vi "차선인식2subVI.vi"(0 "Image In":T9, 1 "Color Mode (Color Threshold 1)":u16(ring) items=["RGB", "HSL", "HSV", "HSI"], 2 "Red or Hue Range (Color Threshold 1)":cluster{"Lower value":i32, "Upper value":i32}={"Lower value"=17, "Upper value"=214}, 3 "Green or Sat Range (Color Threshold 1)":cluster{"Lower value":i32, "Upper value":i32}={"Lower value"=35, "Upper value"=255}, 4 "Blue or Luma or Val or Inten Range (Color Threshold 1)":cluster{"Lower value":i32, "Upper value":i32}={"Lower value"=38, "Upper value"=178}, 5 "Filter Parameters (Filters 1)":T5={"Sigma"=2.0, "HThresh"=0.95, "LThres"=0.8, "WindowSize"=7}, 6 "Operation (Gray Morphology 1)":T4(ring)=enum."Dilate", 7 "error in":errorcluster, 8 "Structuring Element (Gray Morphology 1)":i32[][](array[numeric])=[[1, 1, 1], [1, 1, 1], [1, 1, 1]], 9 "ROI Descriptor (Adv. Straight Edge 1)":T3={"Global Rectangle"=[36, 66, 280, 304], "Contours"=[{"ID"=enum."External", "Type"=12, "Coordinates"=[117, 56, 199, 314, 313366]}]} {"Contours"."Type" items=["No Selection", "Point", "Line", "Rectangle", "Oval", "Polygon", "Freehand Region", "Annulus", "Unused2", "Unused3", "Broken Line", "Freehand Line", "Rotated Rectangle"]}, 10 "Edge Options (Adv. Straight Edge 1)":T2={"Edge Polarity"=1, "Kernel Size"=13, "Width"=3, "Minimum Edge Strength"=26.34, "Interpolation Type"=enum."Zero Order", "Data Processing Method"=enum."Average"} {"Edge Polarity" items=["All Edges", "Rising Edges", "Falling Edges"]}, 11 "Search Direction (Adv. Straight Edge 1)":u32(ring)=1 items=["Left to Right", "Right to Left", "Top to Bottom", "Bottom to Top"], 12 "Line Options (Adv. Straight Edge 1)":T1={"Number of Lines"=1, "Type"=enum."Best Edge Projection", "Min. Score"=0.0, "Max. Score"=1024.0, "Orientation"=0.0, "Angle Range"=20.0, "Angle Tolerance"=1.0, "Step Size"=12, "Min. SNR (db)"=0.0, "Min. Points (%)"=25.0, "Hough Iterations"=5}, 13 "ROI Descriptor (Adv. Straight Edge 2)":T3={"Global Rectangle"=[252, 97, 418, 305], "Contours"=[{"ID"=enum."External", "Type"=12, "Coordinates"=[296, 104, 374, 298, 30219]}]} {"Contours"."Type" items=["No Selection", "Point", "Line", "Rectangle", "Oval", "Polygon", "Freehand Region", "Annulus", "Unused2", "Unused3", "Broken Line", "Freehand Line", "Rotated Rectangle"]}, 14 "Edge Options (Adv. Straight Edge 2)":T2={"Edge Polarity"=1, "Kernel Size"=7, "Width"=3, "Minimum Edge Strength"=122.7, "Interpolation Type"=enum."Zero Order", "Data Processing Method"=enum."Average"} {"Edge Polarity" items=["All Edges", "Rising Edges", "Falling Edges"]}, 15 "Search Direction (Adv. Straight Edge 2)":u32(ring) items=["Left to Right", "Right to Left", "Top to Bottom", "Bottom to Top"], 16 "Line Options (Adv. Straight Edge 2)":T1={"Number of Lines"=1, "Type"=enum."Best Edge Projection", "Min. Score"=0.0, "Max. Score"=1024.0, "Orientation"=0.0, "Angle Range"=20.0, "Angle Tolerance"=1.0, "Step Size"=31, "Min. SNR (db)"=0.0, "Min. Points (%)"=25.0, "Hough Iterations"=5}) -> (20 "Image Out":T9, 21 "Straight Edges (Adv. Straight Edge 1)":T7(array[cluster]) {"Point2 (Real-World)"."Y" format="%.2f"; "Point2 (Real-World)"."X" format="%.2f"; "Point1 (Real-World)"."Y" format="%.2f"; "Point1 (Real-World)"."X" format="%.2f"; "Point2 (Pixels)"."Y" format="%.2f"; "Point2 (Pixels)"."X" format="%.2f"; "Point1 (Pixels)"."Y" format="%.2f"; "Point1 (Pixels)"."X" format="%.2f"}, 22 "Search Lines Information (Adv. Straight Edge 1)":T8(array[cluster]) {"Edges"."Distance (Real-World)" format="%.2f"; "Edges"."Location (Real-World)"."Y" format="%.2g"; "Edges"."Location (Real-World)"."X" format="%.2f"; "Edges"."Noise" format="%.2f"; "Edges"."Location (Pixel)"."Y" format="%.2g"; "Edges"."Location (Pixel)"."X" format="%.2f"; "Edges"."Strength" format="%.2f"; "Edges"."Distance (Pixel)" format="%.2f"; "End Point"."Y" format="%.2f"; "End Point"."X" format="%.2f"; "Start Point"."Y" format="%.2f"; "Start Point"."X" format="%.2f"}, 23 "Used Edges (Adv. Straight Edge 1)":cluster{"Edge Information":T6[]}[](array[cluster]) {"Edge Information"."Distance (Real-World)" format="%.2f"; "Edge Information"."Location (Real-World)"."Y" format="%.2g"; "Edge Information"."Location (Real-World)"."X" format="%.2f"; "Edge Information"."Noise" format="%.2f"; "Edge Information"."Location (Pixel)"."Y" format="%.2g"; "Edge Information"."Location (Pixel)"."X" format="%.2f"; "Edge Information"."Strength" format="%.2f"; "Edge Information"."Distance (Pixel)" format="%.2f"}, 24 "Straight Edges (Adv. Straight Edge 2)":T7(array[cluster]) {"Point2 (Real-World)"."Y" format="%.2f"; "Point2 (Real-World)"."X" format="%.2f"; "Point1 (Real-World)"."Y" format="%.2f"; "Point1 (Real-World)"."X" format="%.2f"; "Point2 (Pixels)"."Y" format="%.2f"; "Point2 (Pixels)"."X" format="%.2f"; "Point1 (Pixels)"."Y" format="%.2f"; "Point1 (Pixels)"."X" format="%.2f"}, 25 "Search Lines Information (Adv. Straight Edge 2)":T8(array[cluster]) {"Edges"."Distance (Real-World)" format="%.2f"; "Edges"."Location (Real-World)"."Y" format="%.2g"; "Edges"."Location (Real-World)"."X" format="%.2f"; "Edges"."Noise" format="%.2f"; "Edges"."Location (Pixel)"."Y" format="%.2g"; "Edges"."Location (Pixel)"."X" format="%.2f"; "Edges"."Strength" format="%.2f"; "Edges"."Distance (Pixel)" format="%.2f"; "End Point"."Y" format="%.2f"; "End Point"."X" format="%.2f"; "Start Point"."Y" format="%.2f"; "Start Point"."X" format="%.2f"}, 26 "Used Edges (Adv. Straight Edge 2)":cluster{"Edge Information":T6[]}[](array[cluster]) {"Edge Information"."Distance (Real-World)" format="%.2f"; "Edge Information"."Location (Real-World)"."Y" format="%.2g"; "Edge Information"."Location (Real-World)"."X" format="%.2f"; "Edge Information"."Noise" format="%.2f"; "Edge Information"."Location (Pixel)"."Y" format="%.2g"; "Edge Information"."Location (Pixel)"."X" format="%.2f"; "Edge Information"."Strength" format="%.2f"; "Edge Information"."Distance (Pixel)" format="%.2f"}, 27 "error out":errorcluster)   [LabVIEW 2020]
uses:
  <vilib>/vision/Image Controls.llb/IMAQ Image.ctl
  <vilib>/vision/Measure.llb/Edge New.ctl
  <vilib>/vision/NI_Vision_Development_Module.lvlib
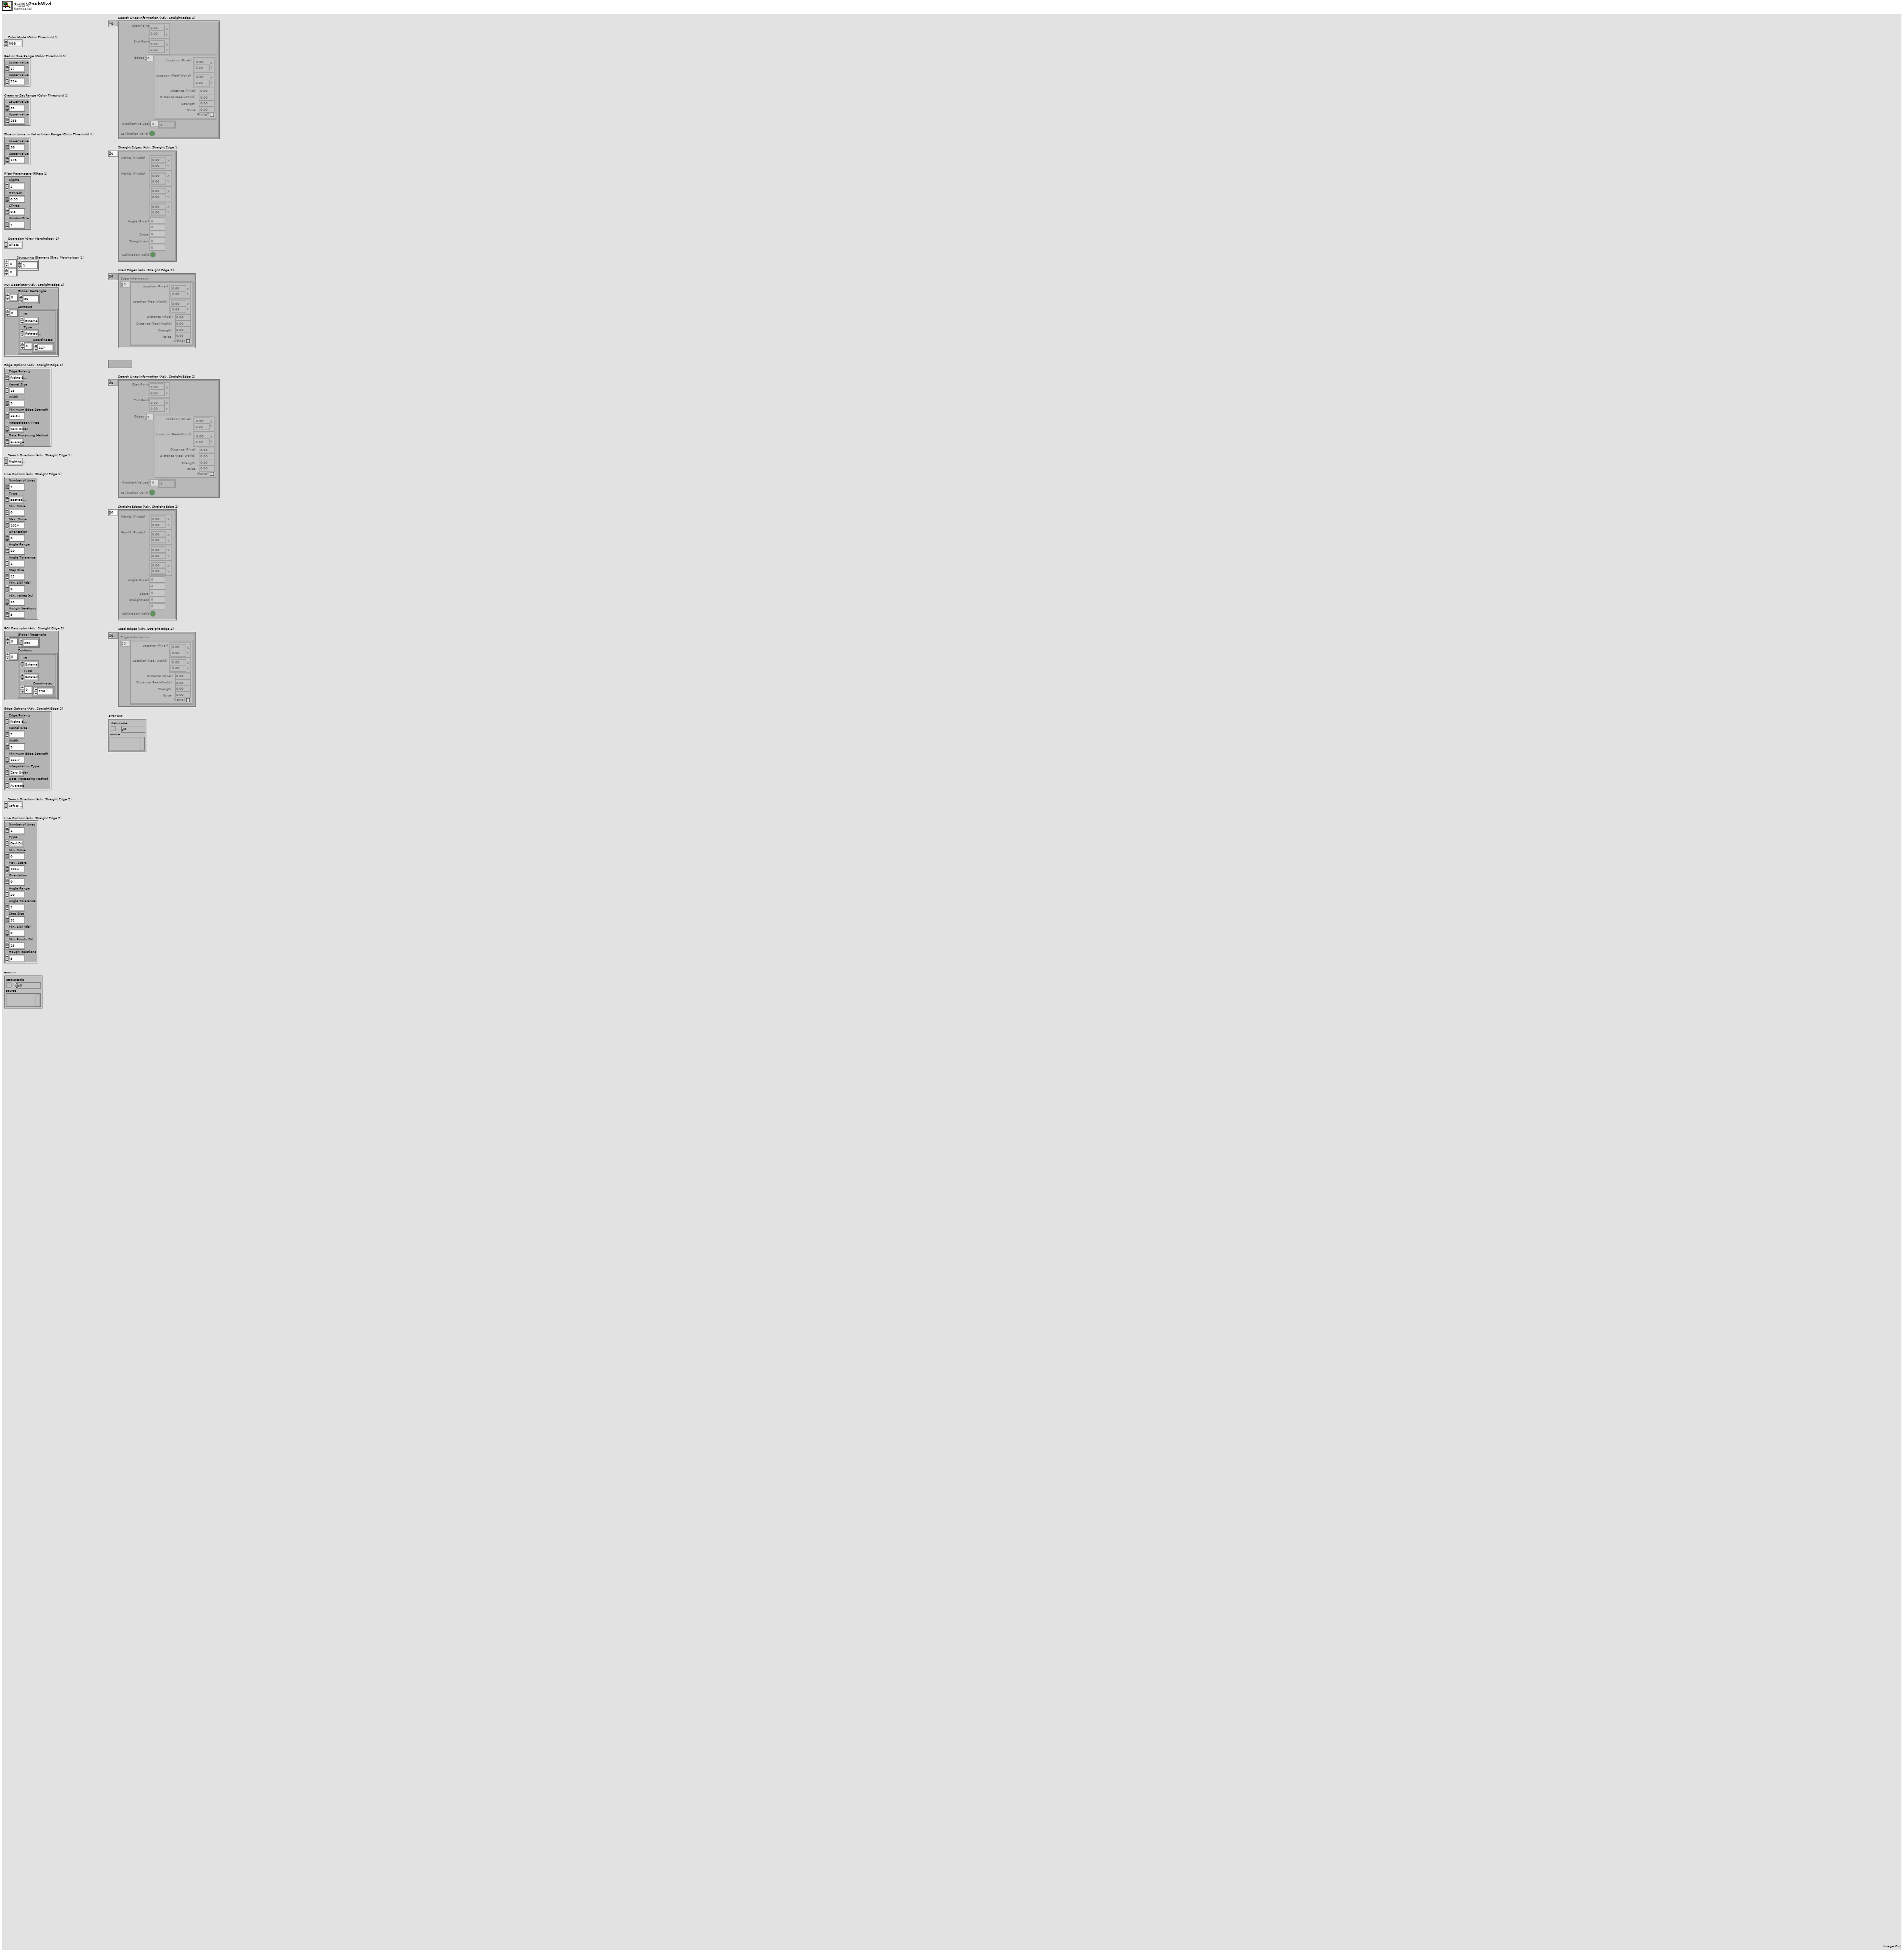
[diagram p1: front panel]
types:
  T1 = cluster{"Number of Lines":i32, "Type":enum32{"First Edge Rake", "Best Edge Rake", "Hough Edge Rake", "First Edge Projection", "Best Edge Projection"}, "Min. Score":dbl, "Max. Score":dbl, "Orientation":dbl, "Angle Range":dbl, "Angle Tolerance":dbl, "Step Size":u32, "Min. SNR (db)":dbl, "Min. Points (%)":dbl, "Hough Iterations":i32}
  T2 = cluster{"Edge Polarity":u32, "Kernel Size":u32, "Width":u32, "Minimum Edge Strength":sgl, "Interpolation Type":enum32{"Zero Order", "Bilinear", "Quadratic", "Cubic", "Bilinear Fixed"}, "Data Processing Method":enum32{"Average", "Median"}}
  T3 = cluster{"Global Rectangle":i32[], "Contours":cluster{"ID":enum32{"External", "Internal"}, "Type":u32, "Coordinates":i32[]}[]}
  T4 = enum32{"AutoM", "Close", "Dilate", "Erode", "Gradient", "Gradient in", "Gradient out", "HitMiss", "Open", "PClose", "POpen", "Thick", "Thin"}
  T5 = cluster{"Sigma":sgl, "HThresh":sgl, "LThres":sgl, "WindowSize":i32}
  T6 = typedef "Edge New.ctl" = cluster{"Location (Pixel)":cluster{"X":sgl, "Y":sgl}, "Location (Real-World)":cluster{"X":sgl, "Y":sgl}, "Distance (Pixel)":dbl, "Distance (Real-World)":dbl, "Strength":dbl, "Noise":dbl, "Rising?":bool}
  T7 = cluster{"Point1 (Pixels)":cluster{"X":sgl, "Y":sgl}, "Point2 (Pixels)":cluster{"X":sgl, "Y":sgl}, "Point1 (Real-World)":cluster{"X":sgl, "Y":sgl}, "Point2 (Real-World)":cluster{"X":sgl, "Y":sgl}, "Angle (Pixel)":dbl, "Angle (Real-World)":dbl, "Score":dbl, "Straightness":dbl, "Average SNR (db)":dbl, "Calibration Valid":bool}[]
  T8 = cluster{"Start Point":cluster{"X":sgl, "Y":sgl}, "End Point":cluster{"X":sgl, "Y":sgl}, "Edges":T6[], "Gradient Values":dbl[], "Calibration Valid":bool}[]
  T9 = typedef "IMAQ Image.ctl" = refnum<image>
  T10 = cluster{"Show Search Area":bool, "Show Search Lines":bool, "Show Edges Found":bool, "Show Result":bool}
  T11 = typedef "Search Line.ctl" = cluster{"Start Point":cluster{"X":sgl, "Y":sgl}, "End Point":cluster{"X":sgl, "Y":sgl}, "Edge Info":T6[], "Edge Map":dbl[], "Calibration Valid":bool}
  T12 = cluster{"Straight Edges":cluster{"Point1 (Pixels)":cluster{"X":sgl, "Y":sgl}, "Point2 (Pixels)":cluster{"X":sgl, "Y":sgl}, "Point1 (Real-World)":cluster{"X":sgl, "Y":sgl}, "Point2 (Real-World)":cluster{"X":sgl, "Y":sgl}, "Angle (Pixel)":dbl, "Angle (Real-World)":dbl, "Score":dbl, "Straightness":dbl, "Average SNR (db)":dbl, "Calibration Valid":bool}[], "Search Lines Information":T11[], "Used Edges":cluster{"Edge Information":T6[]}[]}
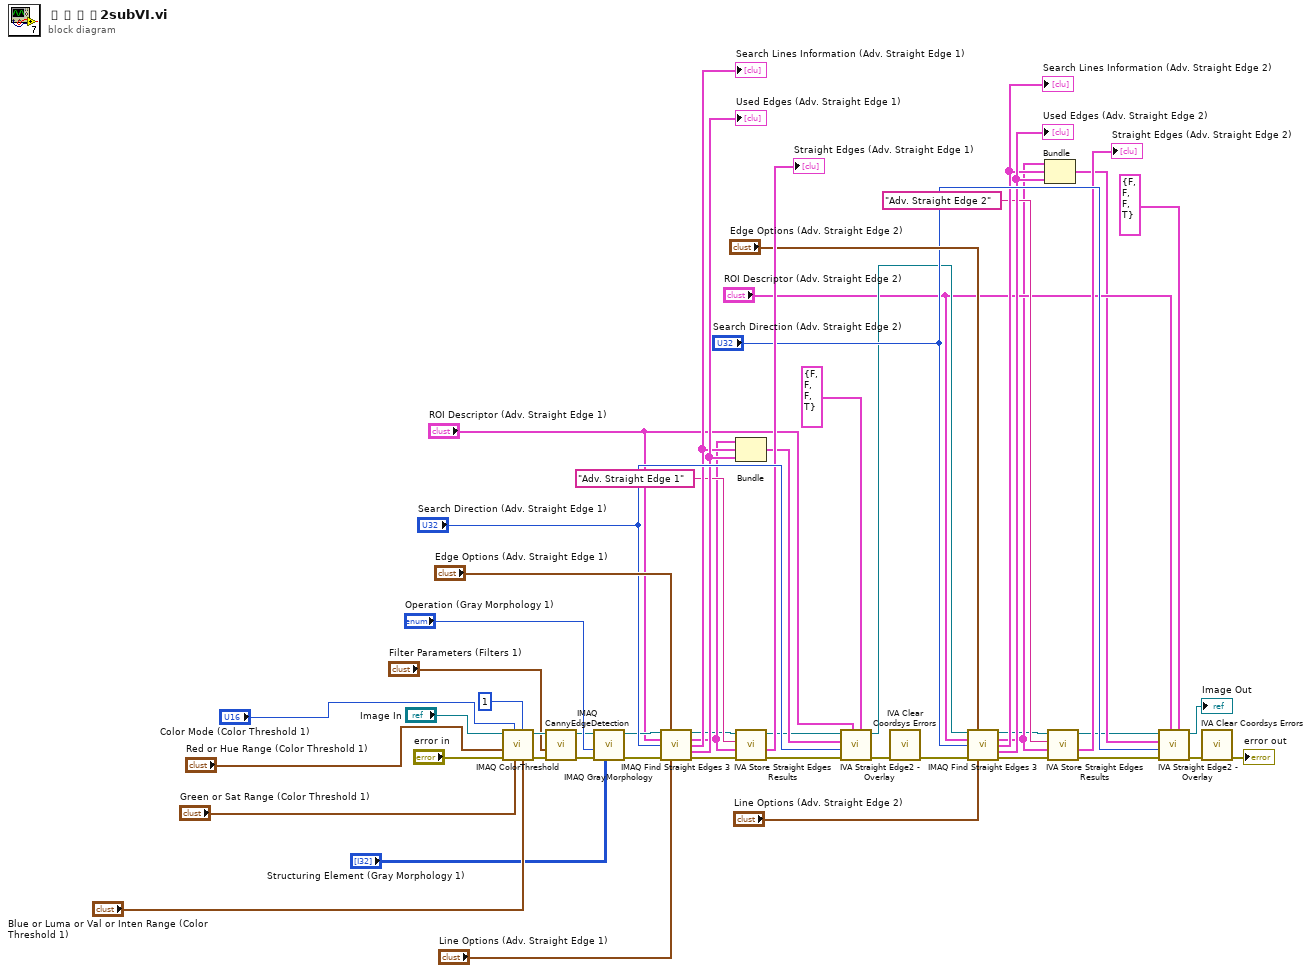
[diagram p0: block diagram]
diagram:
  n1 = call "IMAQ ColorThreshold"("Blue or Luma or Val or Inten Range"="Blue or Luma or Val or Inten Range (Color Threshold 1)", "Replace Value"=1, "Green or Sat Range"="Green or Sat Range (Color Threshold 1)", "Color Mode"="Color Mode (Color Threshold 1)", "error in (no error)"="error in", "Red or Hue Range"="Red or Hue Range (Color Threshold 1)", "Image Src"="Image In") -> ("error out"=w45:errorcluster, "Image Dst Out"=w44:T9)  [unwired: 1 in, 2 out]
  n2 = call "IMAQ CannyEdgeDetection"("Image Src"=w44, "Filter Parameters"="Filter Parameters (Filters 1)", "error in (no error)"=w45) -> ("Image Dst Out"=w39:T9, "error out"=w43:errorcluster)  [unwired: 1 in, 4 out]
  n3 = call "IMAQ GrayMorphology"("Structuring Element"="Structuring Element (Gray Morphology 1)", "error in (no error)"=w43, "Operation"="Operation (Gray Morphology 1)", "Image Src"=w39) -> ("error out"=w38:errorcluster, "Image Dst Out"=w34:T9)  [unwired: 3 in, 3 out]
  n4 = call "IMAQ Find Straight Edges 3"("Image"=w34, "Edge Options"="Edge Options (Adv. Straight Edge 1)", "ROI Descriptor"="ROI Descriptor (Adv. Straight Edge 1)", "Search Direction"="Search Direction (Adv. Straight Edge 1)", "error in (no error)"=w38, "Line Options"="Line Options (Adv. Straight Edge 1)") -> ("Image (duplicate)"=w25:T9, "Straight Edges"=w26:T7, "Search Lines Information"=w31:T11[], "Used Edges"=w32:cluster{"Edge Information":T6[]}[], "error out"=w23:errorcluster)  [unwired: 1 in, 4 out]
  "Search Lines Information (Adv. Straight Edge 1)" <- w31
  "Used Edges (Adv. Straight Edge 1)" <- w32
  n5 = Bundle("Straight Edges"=w26, "Search Lines Information"=w31, "Used Edges"=w32) -> (w27:T12)  [unwired: 1 out]
  n6 = call <vilib>:"IVA Store Straight Edges Results.vi"("error in (no error)"=w23, "Straight Edges"=w26, "Step Name"="Adv. Straight Edge 1", "Image in"=w25) -> ("error out"=w22:errorcluster, "Straight Edges dup"=→"Straight Edges (Adv. Straight Edge 1)":T7, "Image dup"=w24:T9)  [unwired: 5 out]
  n7 = call <vilib>:"IVA Straight Edge2 - Overlay.vi"("Setup"=T10 {"Show Search Area"=FALSE, "Show Search Lines"=FALSE, "Show Edges Found"=FALSE, "Show Result"=TRUE}, "Search Area"="ROI Descriptor (Adv. Straight Edge 1)", "error in (no error)"=w22, "Scan Direction"="Search Direction (Adv. Straight Edge 1)", "Edge Results"=w27, "Image In"=w24) -> ("error out"=w21:errorcluster, "Image Out"=w16:T9)  [unwired: 1 in, 3 out]
  n8 = call <vilib>:"IVA Clear Coordsys Errors.vi"("error in (no error)"=w21) -> ("error out"=w20:errorcluster)  [unwired: 10 in]
  n9 = call "IMAQ Find Straight Edges 3"("Image"=w16, "Edge Options"="Edge Options (Adv. Straight Edge 2)", "ROI Descriptor"="ROI Descriptor (Adv. Straight Edge 2)", "Search Direction"="Search Direction (Adv. Straight Edge 2)", "error in (no error)"=w20, "Line Options"="Line Options (Adv. Straight Edge 2)") -> ("Image (duplicate)"=w6:T9, "Straight Edges"=w7:T7, "Search Lines Information"=w12:T11[], "Used Edges"=w13:cluster{"Edge Information":T6[]}[], "error out"=w4:errorcluster)  [unwired: 1 in, 4 out]
  "Search Lines Information (Adv. Straight Edge 2)" <- w12
  "Used Edges (Adv. Straight Edge 2)" <- w13
  n10 = Bundle("Straight Edges"=w7, "Search Lines Information"=w12, "Used Edges"=w13) -> (w8:T12)  [unwired: 1 out]
  n11 = call <vilib>:"IVA Store Straight Edges Results.vi"("error in (no error)"=w4, "Straight Edges"=w7, "Step Name"="Adv. Straight Edge 2", "Image in"=w6) -> ("error out"=w3:errorcluster, "Straight Edges dup"=→"Straight Edges (Adv. Straight Edge 2)":T7, "Image dup"=w5:T9)  [unwired: 5 out]
  n12 = call <vilib>:"IVA Straight Edge2 - Overlay.vi"("Setup"=T10 {"Show Search Area"=FALSE, "Show Search Lines"=FALSE, "Show Edges Found"=FALSE, "Show Result"=TRUE}, "Search Area"="ROI Descriptor (Adv. Straight Edge 2)", "error in (no error)"=w3, "Scan Direction"="Search Direction (Adv. Straight Edge 2)", "Edge Results"=w8, "Image In"=w5) -> ("error out"=w2:errorcluster, "Image Out"=→"Image Out":T9)  [unwired: 1 in, 3 out]
  n13 = call <vilib>:"IVA Clear Coordsys Errors.vi"("error in (no error)"=w2) -> ("error out"=→"error out":errorcluster)  [unwired: 10 in]
